vi "Read Frequency.vi"(11 "Power Meter in":refnum<class "Power Meter.lvclass">) -> (2 "Frequency":dbl, 3 "Power Meter out":refnum<class "Power Meter.lvclass">)   [LabVIEW 2020, in "Power Meter.lvclass"]
uses:
  Power Meter.lvclass
  Power Meter.lvclass/Power Meter.ctl
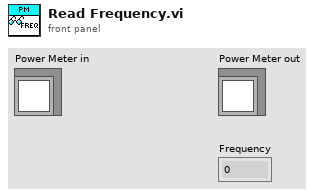
[diagram p1: front panel]
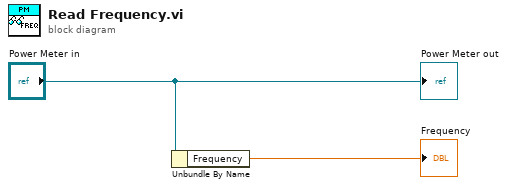
[diagram p0: block diagram]
diagram:
  n1 = Unbundle By Name("Power Meter in") -> ("Frequency"=→"Frequency":dbl)
  "Power Meter out" <- "Power Meter in"
